vi "initHardwareList.vi"(8 "error in (no error)":errorcluster, 10 "HardwareList out":refnum<class "HWConfiguration.lvclass">, 11 "AtomChipHWC in":refnum<class "AtomChipHWC.lvclass">) -> (0 "error out":errorcluster, 3 "AtomChipHWC out":refnum<class "AtomChipHWC.lvclass">)   [LabVIEW 2011, in "Hardware.lvlib" / "HWControllers.lvlib" / "AtomChipHWC.lvclass"]
doc: "initialise hardware list."
uses:
  AtomChipHWC.lvclass
  HardwareConfiguration/HWConfiguration.lvclass
  AtomChipHWC.lvclass/AtomChipHWC.ctl
  HWController.lvclass
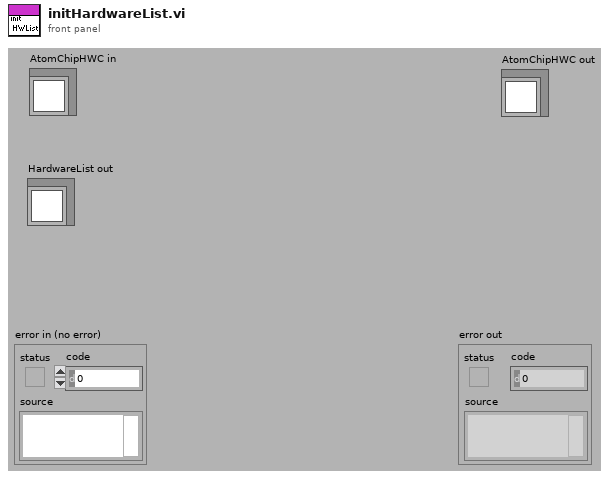
[diagram p1: front panel]
types:
  T1 = enum16{"BEC1", "BEC2", "SingleAtom", "Testing", "AtomChip"}
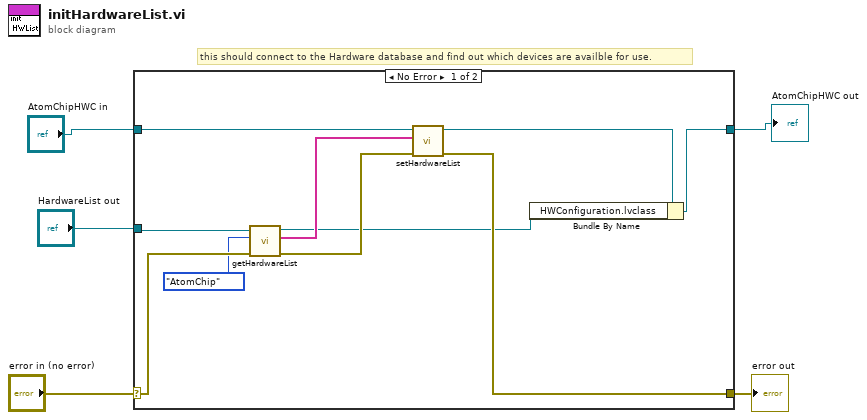
[diagram p0: block diagram]
diagram:
  # "this should connect to the Hardware database and find out which devices are availble for use."
  n1 = case shown="No Error" "error in (no error)" {
    selector: "error in (no error)" -> [w7 w17]
    tunnel: [w12 w17] -> w4
    tunnel: [w9 w16] -> w2
    tunnel: "AtomChipHWC in" -> [w15 w16]
    tunnel: "HardwareList out" -> [w8 _]
    frame No Error {
      n2 = call "getHardwareList.vi"("error in (no error)"=w7, "Enum"=T1."AtomChip", "HWConfiguration in"=w8) -> ("error out"=w13:errorcluster, "HWList"=w14:string[], "HWConfiguration out"=w11:refnum<class "HWConfiguration.lvclass">)  [unwired: 6 in]
      n3 = call "setHardwareList.vi"("error in (no error)"=w13, "hardwareList"=w14, "HWController in"=w15) -> ("error out"=w12:errorcluster, "HWController out"=w10:refnum<class "AtomChipHWC.lvclass">)  [unwired: 7 in]
      n4 = Bundle By Name(cluster=w10, "HWConfiguration.lvclass"=w11) -> (w9:refnum<class "AtomChipHWC.lvclass">)
    }
    frame Error {
    }
  }
  "error out" <- w4
  "AtomChipHWC out" <- w2
